vi "MB schreiben.vi"(0 "TCP Refnum":refnum<k5>, 5 "Address":u16[](array[numeric]), 7 "Coils":bool[](array[boolean]), 9 "Register":u16[](array[numeric]), 11 "error in":errorcluster, 12 "Aktion":T1) -> (4 "TCP Refnum":refnum<k5>, 10 "Exeption Code":u8[](array[numeric]), 15 "error out":errorcluster)   [LabVIEW 2020, in "ABB-EL3000.lvlib" / "Allgemeine VI.lvlib"]
uses:
  Allgemeine VI.lvlib
  Aktion Modbus schreiben.ctl
  <userlib>/NI Modbus.llb/MB Ethernet Master Query Write Single Register (poly).vi
  <userlib>/NI Modbus.llb/MB Ethernet Master Query Write Single Coil (poly).vi
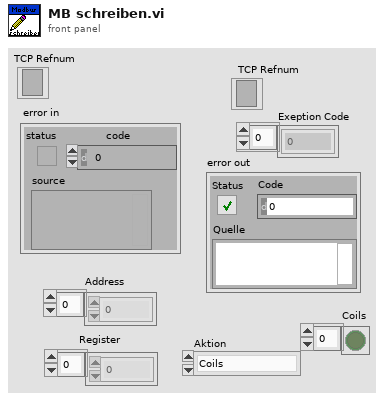
[diagram p1: front panel]
types:
  T1 = typedef "ABB-EL3000.lvlib/Allgemeine VI.lvlib/Aktion Modbus schreiben.ctl" = enum16{"Coils", "Single Register"}
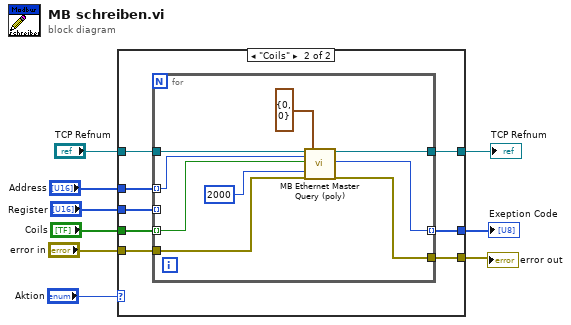
[diagram p0: block diagram]
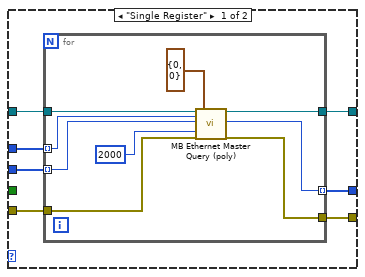
[diagram p2: hidden frame]
diagram:
  n1 = case shown="\"Coils\"" "Aktion" {
    tunnel: "TCP Refnum" -> [w16 w33]
    tunnel: "error in" -> [w15 w32]
    tunnel: [w14 w31] -> w7
    tunnel: "Address" -> [w13 w30]
    tunnel: "Register" -> [w12 w29]
    tunnel: [w11 w28] -> w4
    tunnel: [w10 w27] -> w3
    tunnel: "Coils" -> [_ w26]
    frame "Single Register" {
      n2 = for {
        tunnel: w16 -> [w25]
        tunnel: w15 -> [w24]
        tunnel: [w21] -> w14
        tunnel: w13 -> [w20] mode=indexing
        tunnel: w12 -> [w19] mode=indexing
        tunnel: [w18] -> w11 mode=indexing
        tunnel: [w17] -> w10
        n3 = call-poly <userlib>:"MB Ethernet Master Query (poly).vi"("TCP Connection Refnum in"=w25, "Address"=w20, "Register"=w19, "Timeout"=u32 2000, "error in"=w24, "MBAP Header"=cluster{"Transaction ID":u16, "Unit ID":u8} {"Transaction ID"=0, "Unit ID"=0}) -> ("TCP Connection Refnum (dup)"=w21:refnum<k5>, "Exception Code"=w18:u8, "error out"=w17:errorcluster)  [unwired: 11 in]
      }
    }
    frame "Coils" {
      n4 = for {
        tunnel: w33 -> [w42]
        tunnel: w32 -> [w41]
        tunnel: [w38] -> w31
        tunnel: w30 -> [w37] mode=indexing
        tunnel: w29 -> [_] mode=indexing
        tunnel: [w36] -> w28 mode=indexing
        tunnel: [w35] -> w27
        tunnel: w26 -> [w34] mode=indexing
        n5 = call-poly <userlib>:"MB Ethernet Master Query (poly).vi"("TCP Connection Refnum in"=w42, "Address"=w37, "Coil"=w34, "Timeout"=u32 2000, "error in"=w41, "MBAP Header"=cluster{"Transaction ID":u16, "Unit ID":u8} {"Transaction ID"=0, "Unit ID"=0}) -> ("TCP Connection Refnum (dup)"=w38:refnum<k5>, "Exception Code"=w36:u8, "error out"=w35:errorcluster)  [unwired: 11 in]
      }
    }
  }
  "TCP Refnum" <- w7
  "Exeption Code" <- w4
  "error out" <- w3
